vi "Shut Down.vi"(8 "error in (no error)":errorcluster, 11 "FPGA VI Reference Out":refnum<k20>) -> ()   [LabVIEW 2024]
uses:
  <vilib>/dex/Flush And Wait Empty Condition.ctl
  <vilib>/Utility/error.llb/Error Cluster From Error Code.vi
  <vilib>/rvi/errors/niLvFpgaAdjustHostInterfaceError.vi
  <vilib>/FPGAPlugInAG/Dynamic/niLvFpga_Close_Dynamic.vi
  <vilib>/rvi/interface/nirviReadWriteControl/nirviReadWriteControl.xnode
  <vilib>/rvi/interface/nirviMethod/nirviMethod.xnode
  <vilib>/rvi/interface/nirviCloseFPGA/nirviCloseFPGA.xnode
  <vilib>/FPGAPlugInAG/Dynamic/niLvFpga_StopFifo_Dynamic.vi
  <vilib>/rvi/errors/niLvFpgaMergeErrorWithErrorCode.vi
  NiFpgaLv.dll
  <vilib>/rvi/interface/Simulation/niFpgaSimulationCallBeginRW.vi
panel:
  in  "output cluster":T1
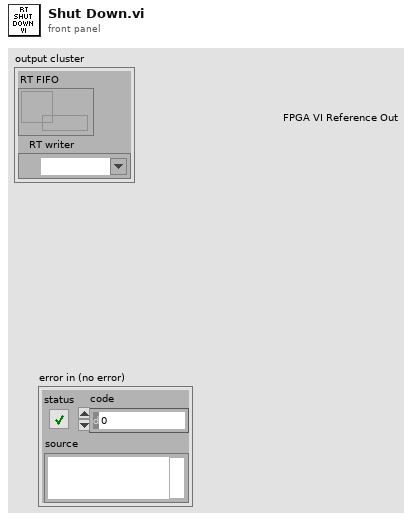
[diagram p1: front panel]
types:
  T1 = cluster{"RT FIFO":refnum<k33>, "RT writer":refnum<k21>}
  T2 = typedef "Flush And Wait Empty Condition.ctl" = u8
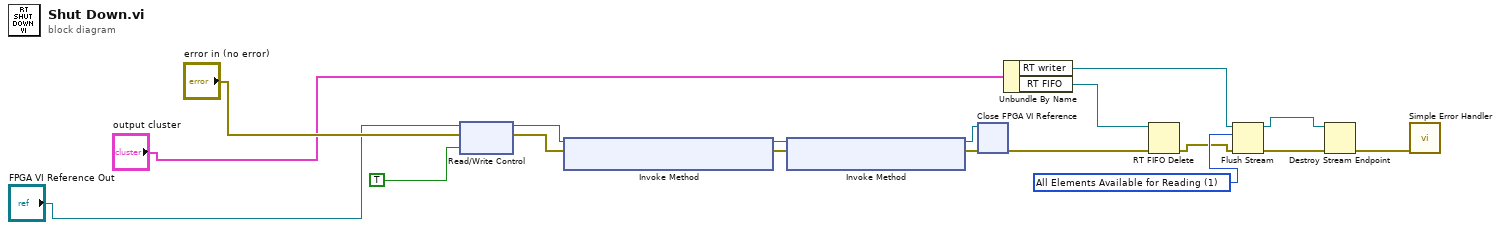
[diagram p0: block diagram]
diagram:
  w15 = T2 1 items=["All Elements Read From Stream", "All Elements Available for Reading"] ("wait condition")
  n1 = xnode "Read/Write Control"("FPGA VI Reference In"="FPGA VI Reference Out", "error in"="error in (no error)", "Stop"=TRUE) -> ("FPGA VI Reference Out"=w3:refnum<k20>, "error out"=w5:errorcluster)
  n2 = xnode "Invoke Method"("FPGA VI Reference In"=w3, "error in"=w5) -> ("FPGA VI Reference Out"=w2:refnum<k20>, "error out"=w4:errorcluster)
  n3 = xnode "Invoke Method"("FPGA VI Reference In"=w2, "error in"=w4) -> ("FPGA VI Reference Out"=w13:refnum<k20>, "error out"=w14:errorcluster)
  n4 = xnode "Close FPGA VI Reference"("FPGA VI Reference In"=w13, "error in"=w14) -> ("error out"=w12:errorcluster)
  n5 = Unbundle By Name("output cluster") -> ("RT writer"=w18:refnum<k21>, "RT FIFO"=w10:refnum<k33>)
  n6 = RT FIFO Delete(0:w10, 3:w12) -> (11:w8:errorcluster)  [unwired: 1 in]
  n7 = Flush Stream(8:w8, 10:w15, 11:w18) -> (0:w7:errorcluster, 3:w16:refnum<k21>)  [unwired: 1 in, 1 out]
  n8 = Destroy Stream Endpoint(8:w7, 11:w16) -> (0:w6:errorcluster)
  n9 = call <vilib>:"Simple Error Handler.vi"("error in (no error)"=w6) -> ()  [unwired: 4 in, 5 out]
